vi "Simple AAP.vi"() -> ()   [LabVIEW 2012]
doc: "该VI可用于采集、分析和演示数据。该VI是LabVIEW核心课程I中练习的答案。步骤信息见教材。"
panel:
  out "平均值":dbl
  out "波形图":dynamicdata(graph)
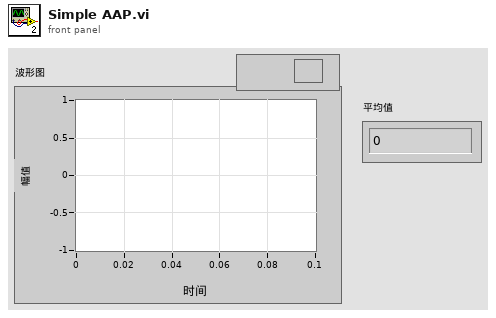
[diagram p1: front panel]
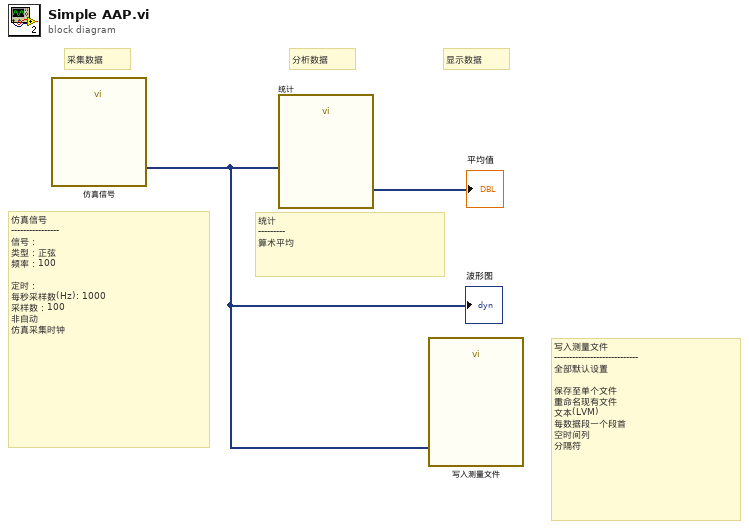
[diagram p0: block diagram]
diagram:
  # "统计\n---------\n算术平均"
  # "写入测量文件\n----------------------------\n全部默认设置\n\n保存至单个文件\n重命名现有文件\n文本(LVM)\n每数据段一个段首\n空时间列\n分隔符"
  # "仿真信号\n----------------\n信号：\n类型：正弦\n频率：100\n\n定时：\n每秒采样数(Hz): 1000\n采样数：100\n非自动\n仿真采集时钟"
  # "显示数据"
  # "分析数据"
  # "采集数据"
  n1 = call "仿真信号"() -> ("正弦"=w2:dynamicdata)  [unwired: 14 in, 1 out]
  "波形图" <- w2
  n2 = call "统计"("Signals"=w2) -> ("Arithmetic Mean"=→"平均值":dynamicdata)  [unwired: 25 in, 1 out]
  n3 = call "写入测量文件"("Signals"=w2) -> ()  [unwired: 16 in, 3 out]
